vi "Write Read Test.vi"(8 "error in (no error)":errorcluster, 10 "Test Value":dbl) -> (0 "error out":errorcluster)   [LabVIEW 2021]
uses:
  Source/Omni-Bus/Omni_Bus.lvclass
  Source/Local Bus/Local Bus.lvclass
  C:/TSA/Omni-Bus/Source/Omni-Bus/Bus Access/Bus_Access.lvclass
  <vilib>/Utility/Data Type/Type Definitions/Data Type.ctl
  <vilib>/TSA/Abstract Data Classes/Abs_Types/Type/Abs_Type.lvclass/Abs_Type.ctl
  Source/Omni-Bus/Omni_Bus.lvclass/Omni_Bus.ctl
  Source/Omni-Bus/Support/Write/Write DBL.vi
  Source/Omni-Bus/Support/Read/Read DBL.vi
  Source/Omni-Bus/Support/FindVar.vi
  <vilib>/Utility/error.llb/Clear Errors.vi
  Source/Omni-Bus/Properties/Read Var Map.vi
  <vilib>/TSA/Abstract Data Classes/Abs_Types/Type/Properties/Read Tag.vi
  <vilib>/TSA/Abstract Data Classes/Abs_Types/Double Float/Abs_Double Float.lvclass
  C:/Program Files (x86)/National Instruments/LabVIEW 2021/vi.lib/TSA/Abstract Data Classes/Abs_Types/Type/Abs_Type.lvclass
  <vilib>/TSA/Abstract Data Classes/Abs_Types/Value/Abs_Value.lvclass
  Source/Omni-Bus/Support/Check For Read Only Error.vi
  Source/Omni-Bus/Support/Incorrect Tag String Error.vi
  <vilib>/addons/_JKI Toolkits/Caraya/classes/Assert/Assert Not Error.vi
  <vilib>/addons/_JKI Toolkits/Caraya/classes/Assert/Assert Equal Value_Variant.vi
  <vilib>/TSA/Abstract Data Classes/Abs_Types/Type/Abs_Type.lvclass
  <vilib>/Utility/Data Type/NI_Data Type.lvlib
  <vilib>/addons/_JKI Toolkits/Caraya/classes/Assert/Assert.lvclass
  <vilib>/addons/_JKI Toolkits/Caraya/classes/Test/Test.lvclass
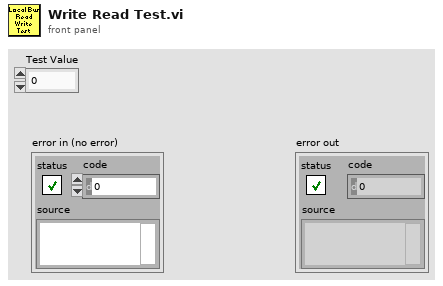
[diagram p1: front panel]
types:
  T1 = typedef "NI_Data Type.lvlib/Data Type.ctl" = enum8{"Invalid Type", "Void", "I8", "I16", "I32", "I64", "U8", "U16", "U32", "U64", "Single Float", "Double Float", "Extended Float", "Single Complex", "Double Complex", "Extended Complex", "Enum U8", "Enum U16", "Enum U32", "Enum U64", "Single Float With Unit", "Double Float With Unit", "Extended Float With Unit", "Single Complex with Unit", "Double Complex with Unit", "Extended Complex with Unit", "Boolean", "String", "Path", "Picture", "Tag", "Array", "Cluster", "Variant", "LV Variant", "Waveform", "Timestamp", "Digital Waveform", "Digital Data", "ExpressData", "Refnum", "External Data", "VI", "Poly VI", "LabVIEW Class Instance", "Fixed Point", "Set Collection", "Map Collection"}
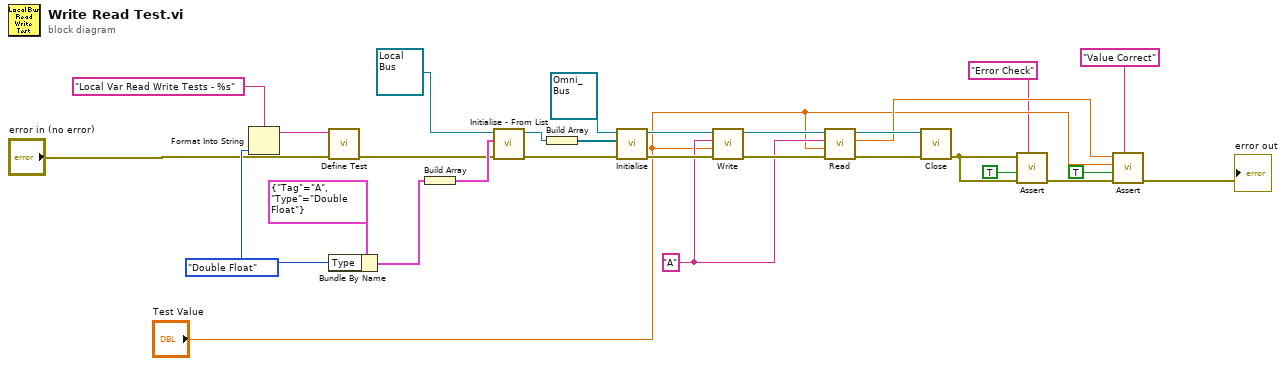
[diagram p0: block diagram]
diagram:
  w10 = Data_Type."Double Float" ("Type")
  w20 = "A" ("Tag")
  n1 = Format Into String(format string="Local Var Read Write Tests - %s", w10) -> (resulting string=w3:string)  [unwired: 2 in, 1 out]
  n2 = call <vilib>:"Define Test.vi"("error in (no error)"="error in (no error)", "Label (VI Title)"=w3) -> ("error out"=w6:errorcluster)  [unwired: 8 in, 1 out]
  n3 = Bundle By Name(cluster=cluster{"Tag":string, "Type":T1} {"Tag"="A", "Type"=enum."Double Float"} ("Cluster"), "Type"=w10) -> (w17:cluster{"Tag":string, "Type":T1})
  n4 = Build Array(w17) -> (w19:cluster{"Tag":string, "Type":T1}[])
  n5 = call "Initialise - From List.vi"("error in (no error)"=w6, "Tag List"=w19, "Local Bus in"=refnum<class "Local Bus.lvclass"> refnum ("Local Bus.lvclass")) -> ("error out"=w27:errorcluster, "Local Bus out"=w28:refnum<class "Local Bus.lvclass">)  [unwired: 7 in]
  n6 = Build Array(w28) -> (w26:refnum<class "Local Bus.lvclass">[])
  n7 = call-dynamic "Initialise.vi"("error in (no error)"=w27, "Bus Access"=w26, "Var Bus in"=refnum<class "Omni_Bus.lvclass"> refnum) -> ("error out"=w21:errorcluster, "Var Bus out"=w22:refnum<class "Omni_Bus.lvclass">)  [unwired: 7 in]
  n8 = call-poly "Write.vi"("error in (no error)"=w21, "Numeric"="Test Value", "Tag"=w20, "Omni_Bus in"=w22) -> ("error out"=w24:errorcluster, "Omni_Bus out"=w23:refnum<class "Omni_Bus.lvclass">)  [unwired: 6 in]
  n9 = call-poly "Read.vi"("error in (no error)"=w24, "Type"="Test Value", "Tag"=w20, "Var Bus in"=w23) -> ("error out"=w15:errorcluster, "Numeric"=w14:dbl, "Var Bus out"=w16:refnum<class "Omni_Bus.lvclass">)  [unwired: 5 in]
  n10 = call-dynamic "Close.vi"("error in (no error)"=w15, "Data in"=w16) -> ("error out"=w4:errorcluster)  [unwired: 8 in, 1 out]
  n11 = call-poly <vilib>:"Assert.vi"("Label"="Error Check", "error in (no error)"=w4, "Register with caller test (F)"=TRUE, "Not Error?"=w4) -> ("error out"=w12:errorcluster)  [unwired: 6 in, 1 out]
  n12 = call-poly <vilib>:"Assert.vi"("Label"="Value Correct", "error in (no error)"=w12, "Register with caller test (F)"=TRUE, "Actual"="Test Value", "Expected"=w14) -> ("error out"=→"error out":errorcluster)  [unwired: 5 in, 1 out]
